vi "CANOpen Export PDO.vi"(8 "error in (no error)":errorcluster, 11 "PDO in":T1[](array[typedef]) {"Bit Offset" max=8 step=1; "Byte Offset" max=8 step=1; "Scale Factor" format="%#_f"}) -> (0 "error out":errorcluster)   [LabVIEW 2021, in "CANOpen Addon System Explorer.lvlib"]
uses:
  CANOpen Addon System Explorer.lvlib
  Shared/CANOpen_PDO Parameter Settings.ctl
  Shared/CANOpen_PDO Data Type.ctl
  Shared/CANopen Byte Order.ctl
  Shared/CANOpen Addon Shared.lvlib
panel:
  out "spreadsheet string":string
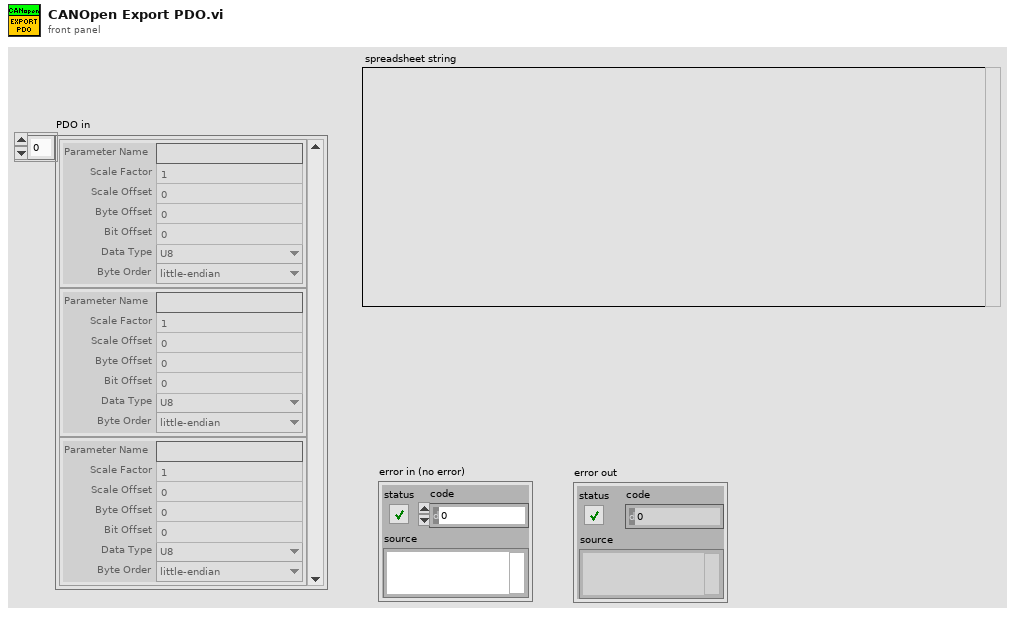
[diagram p1: front panel]
types:
  T1 = typedef "CANOpen Addon Shared.lvlib/CANOpen_PDO Parameter Settings.ctl" = cluster{"Parameter Name":string, "Scale Factor":dbl, "Scale Offset":dbl, "Byte Offset":u8, "Bit Offset":u8, "Data Type":T2, "Byte Order":T3}
  T2 = typedef "CANOpen Addon Shared.lvlib/CANOpen_PDO Data Type.ctl" = enum16{"U8", "U16", "U32", "I8", "I16", "I32", "Single", "Double", "Boolean"}
  T3 = typedef "CANOpen Addon Shared.lvlib/CANopen Byte Order.ctl" = enum16{"big-endian network order", "little-endian"}
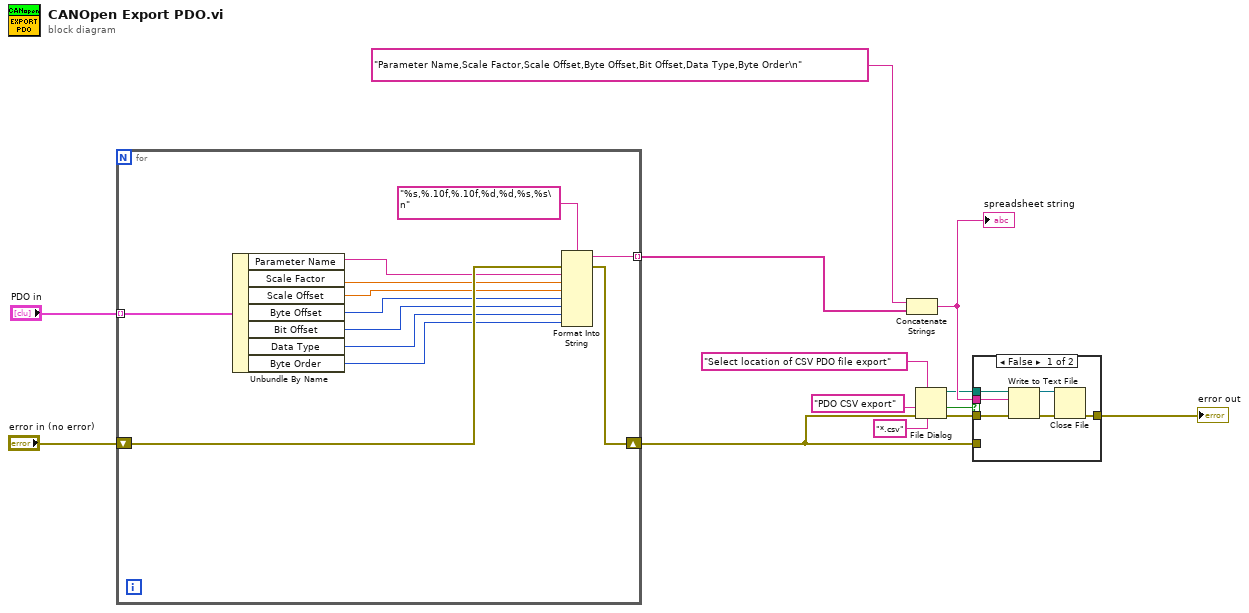
[diagram p0: block diagram]
diagram:
  n1 = for {
    tunnel: "PDO in" -> [w25] mode=indexing
    tunnel: [w22] -> w1 mode=indexing
    shift-right: [w23] -> w2
    shift-left: "error in (no error)" -> [w24]
    n2 = Unbundle By Name(w25) -> ("Parameter Name"=w21:string, "Scale Factor"=w20:dbl, "Scale Offset"=w19:dbl, "Byte Offset"=w18:u8, "Bit Offset"=w17:u8, "Data Type"=w16:T2, "Byte Order"=w15:T3)
    n3 = Format Into String(format string="%s,%.10f,%.10f,%d,%d,%s,%s\n", error in=w24, w21, w20, w19, w18, w17, w16, w15) -> (resulting string=w22:string, error out=w23:errorcluster)  [unwired: 1 in]
  }
  n4 = Concatenate Strings("Parameter Name,Scale Factor,Scale Offset,Byte Offset,Bit Offset,Data Type,Byte Order\n" ("string"), w1) -> (w5:string)
  "spreadsheet string" <- w5
  n5 = File Dialog(6:"*.csv" ("pattern (all files)"), 7:"Select location of CSV PDO file export" ("prompt"), 8:w2, 9:"PDO CSV export" ("default name")) -> (0:w7:errorcluster, 1:w8:bool, 3:w4:path)  [unwired: 3 in, 1 out]
  n6 = case shown="False" w8 {
    tunnel: w7 -> [w31 _]
    tunnel: [w26 w32] -> w6
    tunnel: w2 -> [_ w32]
    tunnel: w5 -> [w30 _]
    tunnel: w4 -> [w29 _]
    frame False {
      n7 = Write to Text File(file (use dialog)=w29, text=w30, error in=w31) -> (refnum out=w27:refnum<file>, error out=w28:errorcluster)  [unwired: 1 in, 1 out]
      n8 = Close File(refnum=w27, error in=w28) -> (error out=w26:errorcluster)  [unwired: 1 out]
    }
    frame True {
    }
  }
  "error out" <- w6
